vi "Lift Core.vi"() -> ()   [LabVIEW 2014]
uses:
  Begin/Global Variables.vi
panel:
  in  "Offset Step":bool
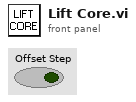
[diagram p1: front panel]
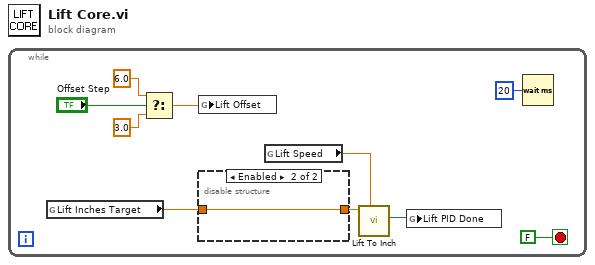
[diagram p0: block diagram]
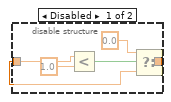
[diagram p2: hidden frame]
diagram:
  n1 = while {
    stop <- FALSE stop-if-true
    n2 = global read "Global Variables.vi" "Lift Inches Target"() -> (w9:dbl)
    n3 = Select(t=6.0, s="Offset Step", f=3.0) -> (s? t:f=w1:dbl)
    n4 = global write "Global Variables.vi" "Lift Offset"(w1) -> ()
    n5 = disable-structure shown="Enabled" {
      disable-tunnel: w9 -> [w12 w16]
      disable-tunnel: [w11 w16] -> w8
      frame Disabled {
        n6 = Less?(x=w12, y=1.0) -> (x < y?=w14:bool)
        n7 = Select(t=0.0, s=w14, f=w12) -> (s? t:f=w11:dbl)
      }
      frame Enabled {
      }
    }
    n8 = global read "Global Variables.vi" "Lift Speed"() -> (w10:dbl)
    n9 = call "Lift To Inch.vi"("Speed"=w10, "Inches to move"=w8) -> ("Done"=w7:bool)  [unwired: 9 in]
    n10 = global write "Global Variables.vi" "Lift PID Done"(w7) -> ()
    n11 = Wait (ms)(milliseconds to wait=u32 20) -> ()  [unwired: 1 out]
  }
